vi "closeFncGen_AS.vi"(1 "error in (no error)":errorcluster, 3 "VISA resource name":refnum<visa-resource-name>="GPIB0::4::INSTR") -> (0 "error out":errorcluster)   [LabVIEW 2016]
doc: "Shows how to configure then create an arbitrary waveform."
uses:
  Agilent 33XXX Series.lvlib
panel:
  # "(c) 2005 - 2013 National Instruments.  ALL RIGHTS RESERVED."
  # "To edit the Arbitrary Waveform, use the Simulate Arbitrary Signal on the block diagram; or choose from the options below."
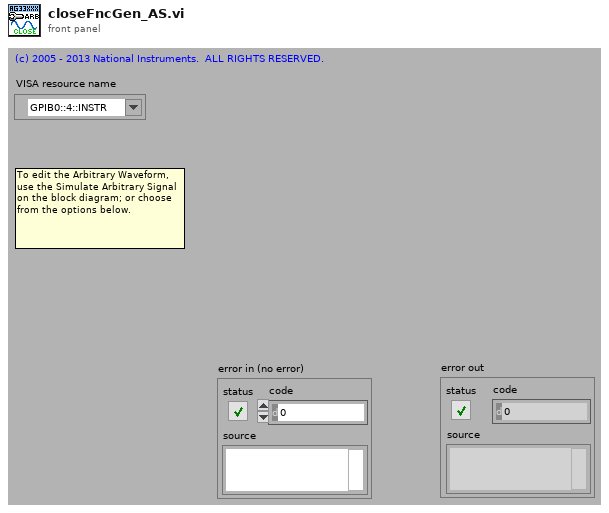
[diagram p1: front panel]
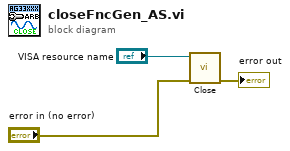
[diagram p0: block diagram]
diagram:
  n1 = call "Close.vi"("error in (no error)"="error in (no error)", "VISA resource name"="VISA resource name") -> ("error out"=→"error out":errorcluster)  [unwired: 9 in]
